vi "Module Loop.vi"(8 "error in (no error)":errorcluster, 11 "Data Logger Module in":refnum<class "Data Logger Module.lvclass">) -> (0 "error out":errorcluster, 3 "Data Logger Module out":refnum<class "Data Logger Module.lvclass">)   [LabVIEW 2020, in "VolatusData.lvlib" / "Data Logger Module.lvclass"]
uses:
  Data Logger Module.lvclass
  C:/dev/lv20CE/relink/lv-volatus/Volatus/Module/Module.lvclass
  Data Logger Module.lvclass/Data Logger Module.ctl
  Volatus/Module/Module.lvclass
  New Data.ctl
  Prepare Log.ctl
  Volatus/Module/Module.lvclass/Module.ctl
  <vilib>/Utility/error.llb/Error Cluster From Error Code.vi
  VolatusData.lvlib
panel:
  out "Parent Name":string
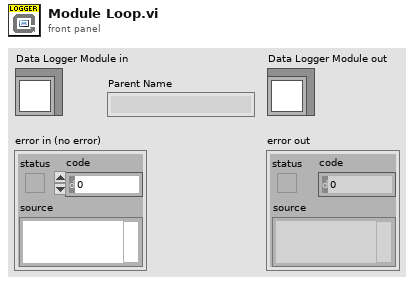
[diagram p1: front panel]
types:
  T1 = typedef "VolatusData.lvlib/New Data.ctl" = cluster{"Channels":waveform(dbl)[]}
  T2 = typedef "VolatusData.lvlib/Prepare Log.ctl" = cluster{"Folder":path, "Series":string}
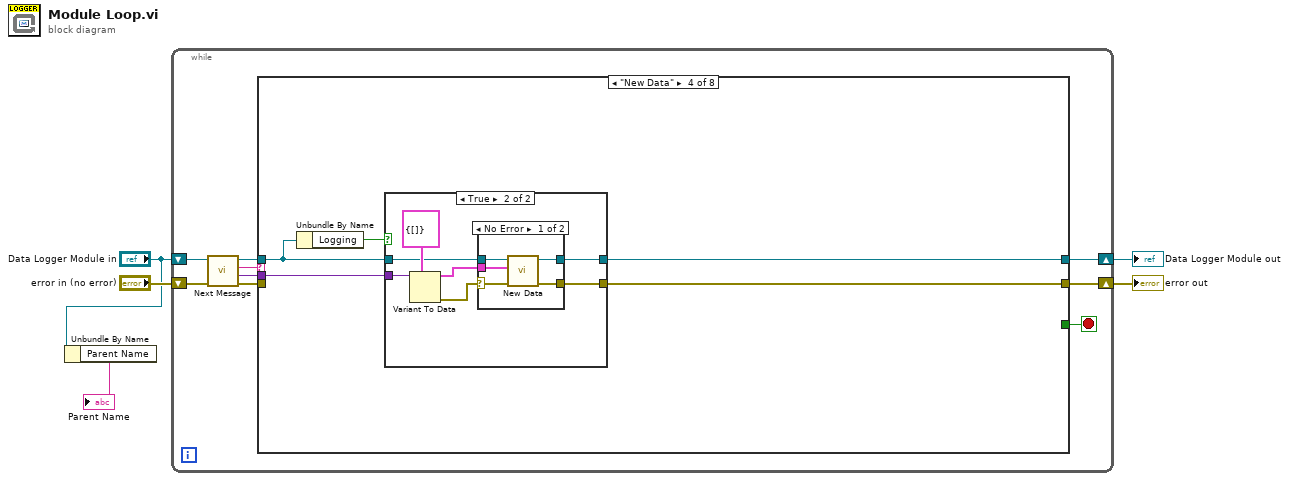
[diagram p0: block diagram]
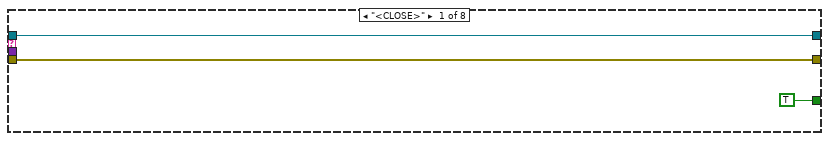
[diagram p2: hidden frame]
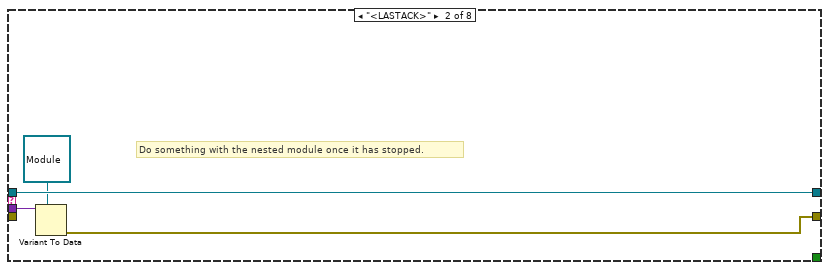
[diagram p3: hidden frame]
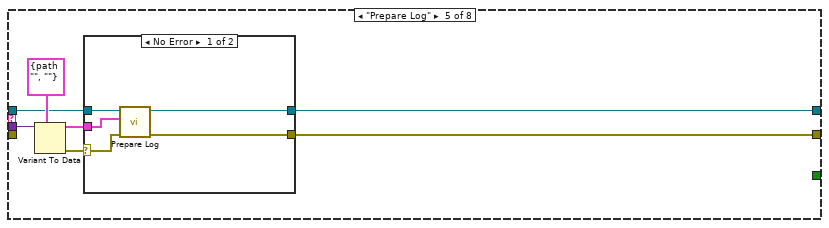
[diagram p7: hidden frame]
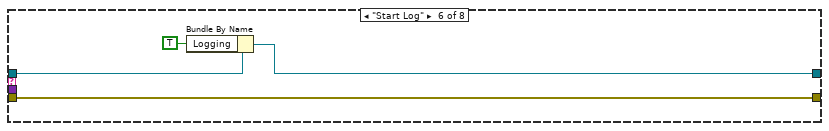
[diagram p9: hidden frame]
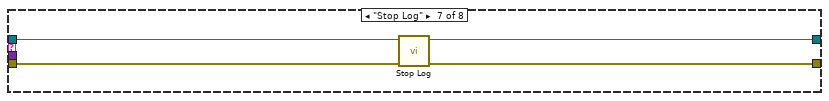
[diagram p10: hidden frame]
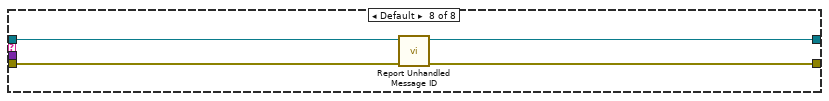
[diagram p11: hidden frame]
diagram:
  n1 = Unbundle By Name("Data Logger Module in") -> ("Parent Name"=→"Parent Name":string)
  n2 = while {
    shift-right: [w9] -> w4
    shift-left: "Data Logger Module in" -> [w14]
    shift-right: [w8] -> w3
    shift-left: "error in (no error)" -> [w13]
    stop <- w7 stop-if-true
    n3 = call "Next Message.vi"("error in (no error)"=w13, "Module in"=w14) -> ("error out"=w12:errorcluster, "Data"=w6:variant, "ID"=w11:string, "Module out"=w10:refnum<class "Data Logger Module.lvclass">)  [unwired: 6 in]
    n4 = case shown="\"New Data\"" w11 {
      tunnel: w12 -> [w15 _ w22 _ _ w60 w65 w69]
      tunnel: w10 -> [w16 w21 w23 w26 w46 w61 w63 w67]
      tunnel: [w16 w21 w23 w25 w45 w59 w62 w66] -> w9
      tunnel: [w15 w18 w22 w24 w44 w60 w64 w68] -> w8
      tunnel: [TRUE _ _ _ _ _ _ _] -> w7
      tunnel: w6 -> [_ w20 _ w28 w50 _ _ _]
      frame "<CLOSE>" {
      }
      frame "<LASTACK>" {
        # "Do something with the nested module once it has stopped."
        n5 = Variant To Data(type=refnum<class "Module.lvclass"> refnum ("Volatus:Module"), Variant=w20) -> (error out=w18:errorcluster)  [unwired: 1 in, 1 out]
      }
      frame "<TIMEOUT>" {
        # "No message for this module was received in time"
      }
      frame "New Data" {
        n6 = Unbundle By Name(w26) -> ("Logging"=w27:bool)
        n7 = case shown="True" w27 {
          tunnel: w28 -> [_ w36]
          tunnel: w26 -> [w29 w34]
          tunnel: [w29 w31] -> w25
          tunnel: [_ w30] -> w24
          frame False {
          }
          frame True {
            n8 = Variant To Data(type=T1 {"Channels"=[]} ("New Data"), Variant=w36) -> (data=w33:T1, error out=w32:errorcluster)  [unwired: 1 in]
            n9 = case shown="No Error" w32 {
              selector: w32 -> [w39 w43]
              tunnel: w34 -> [w41 w42]
              tunnel: w33 -> [w40 _]
              tunnel: [w38 w42] -> w31
              tunnel: [w37 w43] -> w30
              frame No Error {
                n10 = call "New Data.vi"("error in (no error)"=w39, "New Data"=w40, "Data Logger Module in"=w41) -> ("error out"=w37:errorcluster, "Data Logger Module out"=w38:refnum<class "Data Logger Module.lvclass">)  [unwired: 7 in]
              }
              frame Error {
              }
            }
          }
        }
      }
      frame "Prepare Log" {
        n11 = Variant To Data(type=T2 {"Folder"=path "", "Series"=""} ("Prepare Log"), Variant=w50) -> (data=w47:T2, error out=w48:errorcluster)  [unwired: 1 in]
        n12 = case shown="No Error" w48 {
          selector: w48 -> [w53 w56]
          tunnel: w47 -> [w54 _]
          tunnel: w46 -> [w55 w57]
          tunnel: [w52 w57] -> w45
          tunnel: [w51 w56] -> w44
          frame No Error {
            n13 = call "Prepare Log.vi"("error in (no error)"=w53, "Prepare Log"=w54, "Data Logger Module in"=w55) -> ("error out"=w51:errorcluster, "Data Logger Module out"=w52:refnum<class "Data Logger Module.lvclass">)  [unwired: 7 in]
          }
          frame Error {
          }
        }
      }
      frame "Start Log" {
        n14 = Bundle By Name(cluster=w61, "Logging"=TRUE) -> (w59:refnum<class "Data Logger Module.lvclass">)
      }
      frame "Stop Log" {
        n15 = call "Stop Log.vi"("error in (no error)"=w65, "Data Logger Module in"=w63) -> ("error out"=w64:errorcluster, "Data Logger Module out"=w62:refnum<class "Data Logger Module.lvclass">)  [unwired: 8 in]
      }
      frame Default {
        n16 = call "Report Unhandled Message ID.vi"("error in (no error)"=w69, "Module in"=w67) -> ("error out"=w68:errorcluster, "Module out"=w66:refnum<class "Data Logger Module.lvclass">)  [unwired: 8 in]
      }
    }
  }
  "error out" <- w3
  "Data Logger Module out" <- w4
